vi "USB5CloseDevice.vi"(8 "错误输入（无错误）":errorcluster, 11 "DevIndex":i32) -> (0 "error out":errorcluster caption="错误输出", 3 "DevIndex Out":i32)   [LabVIEW 2020]
uses:
  lib/x64/USB5000.dll
panel:
  out "ErrorCode":i32
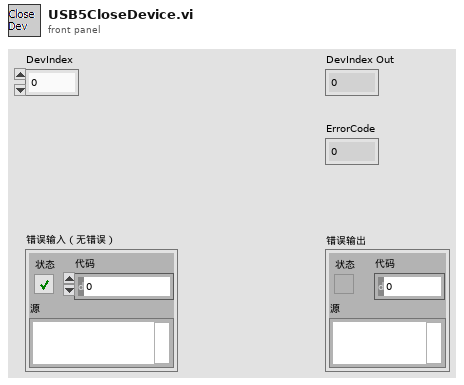
[diagram p1: front panel]
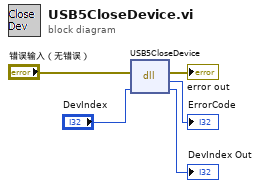
[diagram p0: block diagram]
diagram:
  n1 = dll-call lib="C:/Users/phosense/Downloads/USB-5000/USB-5000_LabVIEW/lib/x64/USB5000.dll" fn="USB5CloseDevice"(error in="错误输入（无错误）", "DevIndex"="DevIndex") -> (error out=→"error out":errorcluster, "返回类型"=→"ErrorCode":i32, "DevIndex"=→"DevIndex Out":i32)  [unwired: 2 in, 1 out]
